vi "Test Trim Whitspace.vi"() -> ()   [LabVIEW 2015, in "JSONtext.lvlib"]
uses:
  JSONtext.lvlib
  <vilib>/Utility/error.llb/whitespace.ctl
  <userlib>/_OpenG.lib/string/string.llb/Trim Whitespace (String)__ogtk.vi
panel:
  in  "dimension size":i32=10
  out "x-y":dbl format="%#_6p"
  out "Array":string[](array[string])
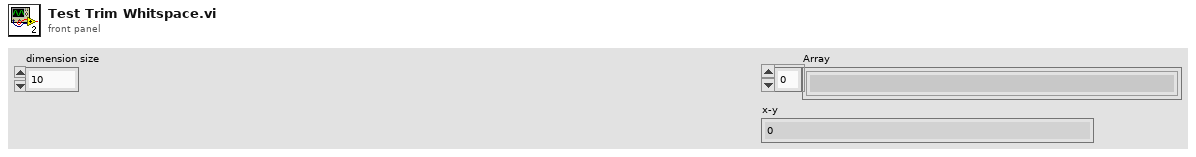
[diagram p1: front panel]
types:
  T1 = typedef "whitespace.ctl" = u16
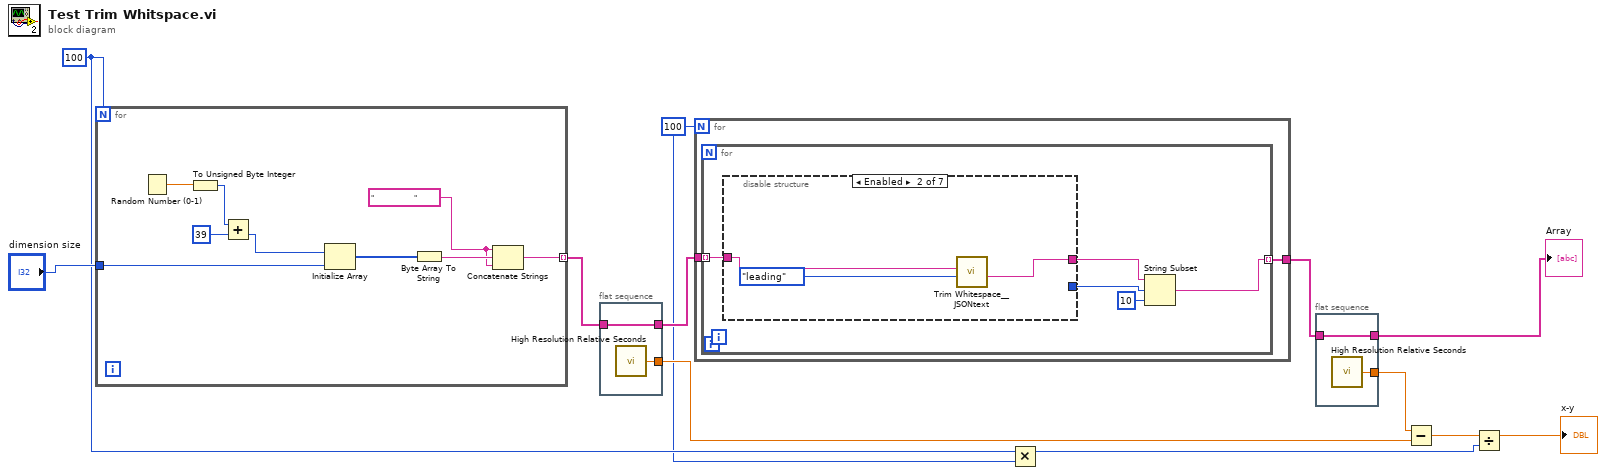
[diagram p0: block diagram]
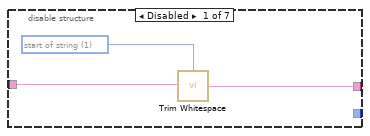
[diagram p2: hidden frame]
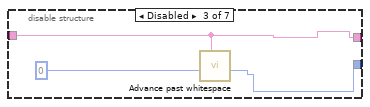
[diagram p3: hidden frame]
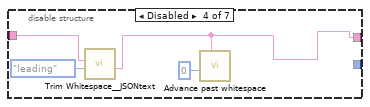
[diagram p4: hidden frame]
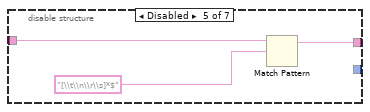
[diagram p5: hidden frame]
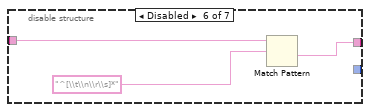
[diagram p6: hidden frame]
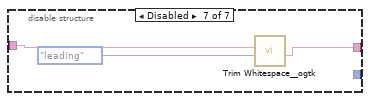
[diagram p7: hidden frame]
diagram:
  w1 = 100
  w4 = 100
  n1 = for {
    N: w4 -> [_]
    tunnel: [w17] -> w12 mode=indexing
    tunnel: "dimension size" -> [w13]
    w18 = "                    " ("element")
    n2 = Random Number (0-1)() -> (number: 0 to 1=w16:dbl)
    n3 = To Unsigned Byte Integer(number=w16) -> (unsigned 8bit integer=w14:u8)
    n4 = Add(x=w14, y=u8 39) -> (x+y=w15:u8)
    n5 = Initialize Array(w15, w13) -> (w20:u8[])
    n6 = Byte Array To String(unsigned byte array=w20) -> (string=w19:string)
    n7 = Concatenate Strings(w18, w19, w18) -> (w17:string)
  }
  n8 = flat-sequence {
    tunnel: [w23] -> w11
    tunnel: w12 -> [w23]
    tunnel: [w22] -> w8
    frame #0 {
      n9 = call <vilib>:"High Resolution Relative Seconds.vi"() -> ("relative seconds"=w22:dbl)
    }
  }
  n10 = for {
    N: w1 -> [_]
    tunnel: w11 -> [w25]
    tunnel: [w24] -> w10
    n11 = for {
      tunnel: w25 -> [w30] mode=indexing
      tunnel: [w28] -> w24 mode=indexing
      n12 = disable-structure shown="Enabled" {
        disable-tunnel: w30 -> [w33 w36 w38 w42 w45 w48 w52]
        disable-tunnel: [w32 w35 w38 w40 w44 w47 w51] -> w29
        disable-tunnel: [_ _ w37 _ _ _ _] -> w26
        frame Disabled {
          w31 = T1 1 items=["both", "start of string", "end of string"] ("location (both)")
          n13 = call <vilib>:"Trim Whitespace.vi"("string"=w33, "location (both)"=w31) -> ("trimmed string"=w32:string)
        }
        frame Enabled {
          n14 = call "Trim Whitespace__JSONtext.vi"("Remove (leading and trailing)"=enum16{"leading", "trailing", "both"}."leading", "String in"=w36) -> ("String out"=w35:string)  [unwired: 5 in]
        }
        frame Disabled {
          n15 = call "Advance past whitespace.vi"("JSON"=w38, "Offset"=0) -> ("Offset of first non-whitespace"=w37:i32)  [unwired: 8 in, 1 out]
        }
        frame Disabled {
          n16 = call "Trim Whitespace__JSONtext.vi"("Remove (leading and trailing)"=enum16{"leading", "trailing", "both"}."leading", "String in"=w42) -> ("String out"=w40:string)  [unwired: 5 in]
          n17 = call "Advance past whitespace.vi"("JSON"=w40, "Offset"=0) -> ()  [unwired: 8 in, 2 out]
        }
        frame Disabled {
          n18 = Match Pattern(string=w45, regular expression="[\\t\\n\\r\\s]*$") -> (before substring=w44:string)  [unwired: 1 in, 3 out]
        }
        frame Disabled {
          n19 = Match Pattern(string=w48, regular expression="^[\\t\\n\\r\\s]*") -> (after substring=w47:string)  [unwired: 1 in, 3 out]
        }
        frame Disabled {
          n20 = call-poly <userlib>:"Trim Whitespace__ogtk.vi"("Remove (leading and trailing)"=enum16{"leading", "trailing", "both"}."leading", "String in"=w52) -> ("String out"=w51:string)  [unwired: 5 in]
        }
      }
      n21 = String Subset(string=w29, offset (0)=w26, length (rest)=10 ("length (rest)")) -> (substring=w28:string)
    }
  }
  n22 = Multiply(x=w4, y=w1) -> (x*y=w2:i32)
  n23 = flat-sequence {
    tunnel: [w54] -> w3
    tunnel: w10 -> [w54]
    tunnel: [w53] -> w9
    frame #0 {
      n24 = call <vilib>:"High Resolution Relative Seconds.vi"() -> ("relative seconds"=w53:dbl)
    }
  }
  n25 = Subtract(x=w9, y=w8) -> (x-y=w7:dbl)
  n26 = Divide(x=w7, y=w2) -> (x/y=→"x-y":dbl)
  "Array" <- w3
